vi "OMA.vi"(0 "System no.":i32=1 min=1 max=4 step=1, 2 "Axes to move":string[](array[string]), 3 "Position values":dbl[](array[numeric]) format="%.6f", 4 "No.of digits":i16=4, 5 "error in":errorcluster) -> (19 "error out":errorcluster)   [LabVIEW 2020]
doc: "Open-loop move absolute. Sets new absolute open-loop target position for given axes. Servo must be disabled for all commanded axes prior to using this command.\n\nE-861: This command works only in open-loop operation. With closed-loop systems, use MOV instead to command motion. Do not call OMA or OMR for axes which have no sensor, otherwise stage will run into hard stop. Motion commands are not allowed when a joystick is active on the axis. OMA can not be processed as long as motion commanded by a former OMA or OMR command is still performed.\n\nE-871, E-873: This command works only in open-loop operation. With closed-loop systems, use MOV instead to command motion. Do not call OMA or OMR for axes which have no sensor, otherwise stage will run into hard stop. Motion commands are not allowed when a joystick is active on the axis."
panel:
  # "Open-loop Move Absolute. Sets new absolute open-loop target \nposition for given axes."
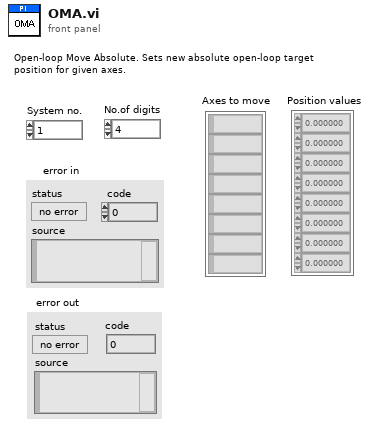
[diagram p1: front panel]
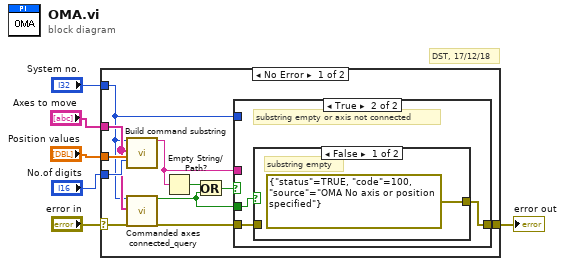
[diagram p0: block diagram]
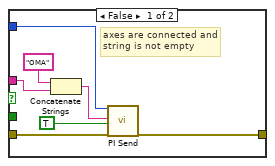
[diagram p2: hidden frame]
diagram:
  # "DST, 17/12/18"
  n1 = case shown="No Error" "error in" {
    selector: "error in" -> [w10 w30]
    tunnel: [w17 w30] -> w6
    tunnel: "Position values" -> [w16 _]
    tunnel: "No.of digits" -> [w15 _]
    tunnel: "System no." -> [w11 _]
    tunnel: "Axes to move" -> [w13 _]
    frame No Error {
      n2 = call "Build command substring.vi"("System no."=w11, "Affected axes"=w13, "Parameters"=w16, "No. of digits"=w15) -> ("Command substring"=w7:string)  [unwired: 3 in, 12 out]
      n3 = call "Commanded axes connected_query.vi"("System no."=w11, "Commanded axes"=w13, "error in"=w10) -> ("Controller error"=w9:bool, "error out"=w14:errorcluster)  [unwired: 1 in, 14 out]
      n4 = Empty String/Path?(string/path=w7) -> (empty?=w8:bool)
      n5 = Or(x=w8, y=w9) -> (x .or. y?=w12:bool)
      n6 = case shown="True" w12 {
        tunnel: w7 -> [w23 _]
        tunnel: [w19 w27] -> w17
        tunnel: w14 -> [w20 w25]
        tunnel: w9 -> [_ w26]
        tunnel: w11 -> [w18 _]
        frame False {
          # "axes are connected and\nstring is not empty"
          n7 = Concatenate Strings("OMA", w23) -> (w21:string)
          n8 = call "PI Send.vi"("System no."=w18, "String to send"=w21, "Attach termination char.?"=TRUE ("Attach Linefeed?"), "error in"=w20) -> ("error out"=w19:errorcluster)  [unwired: 2 in, 13 out]
        }
        frame True {
          # "substring empty or axis not connected"
          n9 = case shown="False" w26 {
            tunnel: [errorcluster {"status"=TRUE, "code"=100, "source"="OMA No axis or position specified"} ("error out") w29] -> w27
            tunnel: w25 -> [_ w29]
            frame False {
              # "substring empty"
            }
            frame True {
              # "commanded axis \nnot connected"
            }
          }
        }
      }
    }
    frame Error {
    }
  }
  "error out" <- w6
